vi "UserInfos.vi"() -> ()   [LabVIEW 2013]
panel:
  in  "UserInfos":T1
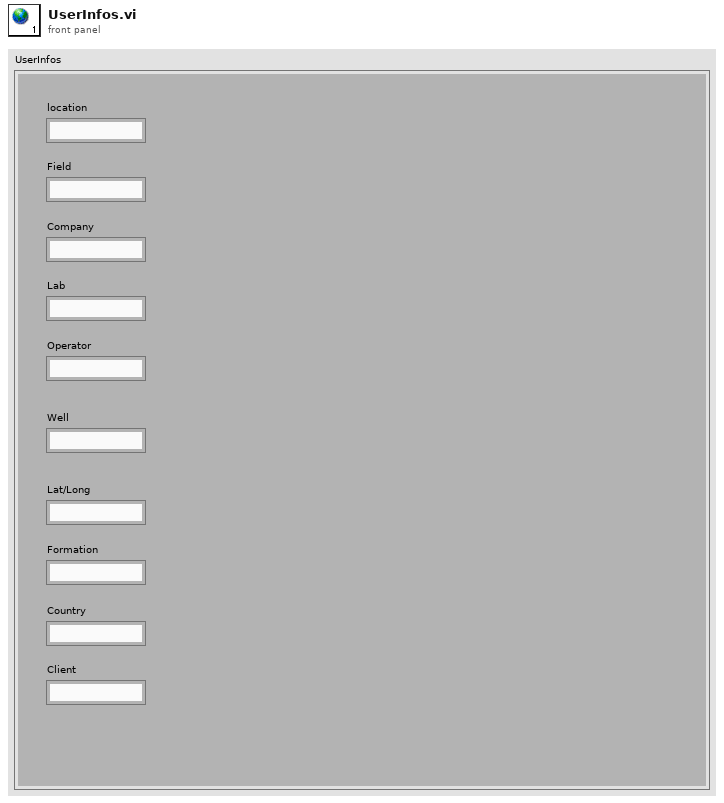
[diagram p1: front panel]
types:
  T1 = cluster{"location":string, "Field":string, "Company":string, "Lab":string, "Operator":string, "Well":string, "Lat/Long":string, "Formation":string, "Country":string, "Client":string}
diagram:
